vi "validate line configuration.vi"(7 "module configuration":refnum<class "Shared Library Module configuration.lvclass">, 11 "line in":T1) -> (1 "valid?":bool, 3 "line out":T1)   [LabVIEW 2013, in "Shared Library Module editor node.lvclass"]
doc: "Platypus Framework 1.0.1.60\nNI Systems Engineering - National Instruments"
uses:
  Shared Library Module editor node.lvclass
  <vilib>/NI/Tag Bus Module Framework/channel/TBM channel.lvclass
  table line.ctl
  configuration/Shared Library Module configuration.lvclass
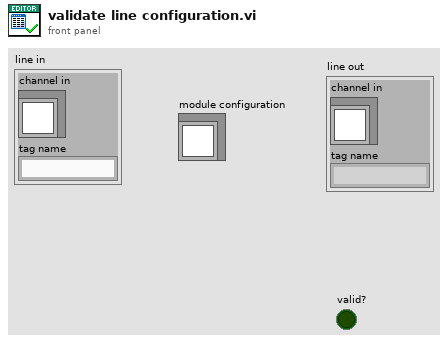
[diagram p1: front panel]
types:
  T1 = typedef "Shared Library Module editor node.lvclass/table line.ctl" = cluster{"channel in":refnum<class "TBM channel.lvclass">, "tag name":string}
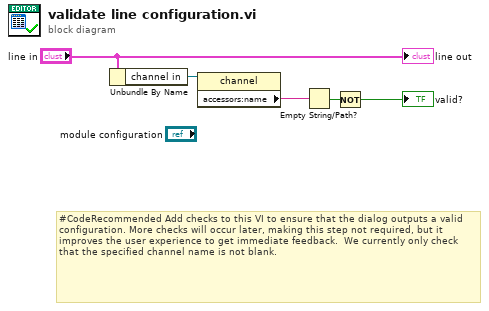
[diagram p0: block diagram]
diagram:
  # "#CodeRecommended Add checks to this VI to ensure that the dialog outputs a valid configuration. More checks will occur later, making this step not required, but it improves the user experience to get immediate feedback.  We currently only check that the specified channel name is not blank."
  n1 = Unbundle By Name("line in") -> ("channel in"=w4:refnum<class "TBM channel.lvclass">)
  n2 = property class="channel"(reference=w4) -> ("accessors:name"=w3:string)  [unwired: 1 in, 2 out]
  n3 = Empty String/Path?(string/path=w3) -> (empty?=w2:bool)
  n4 = Not(x=w2) -> (.not. x?=→"valid?":bool)
  "line out" <- "line in"
